vi "Create.vi"(8 "error in (no error)":errorcluster, 10 "Logging Rate":dbl) -> (0 "error out":errorcluster, 3 "Historian Logger out":refnum<class "Historian Logger.lvclass">)   [LabVIEW 2020, in "VolatusHistorian.lvlib" / "Historian Logger.lvclass"]
uses:
  Historian Logger.lvclass
  Historian Logger.lvclass/Historian Logger.ctl
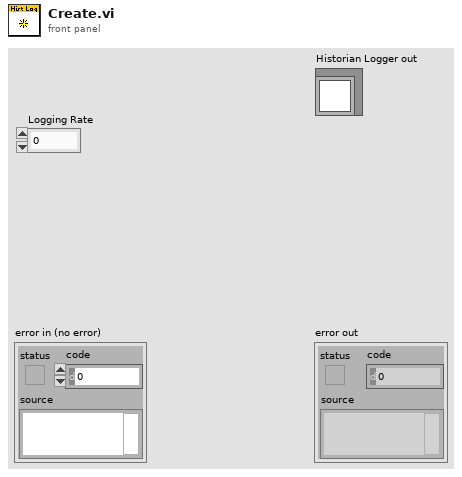
[diagram p1: front panel]
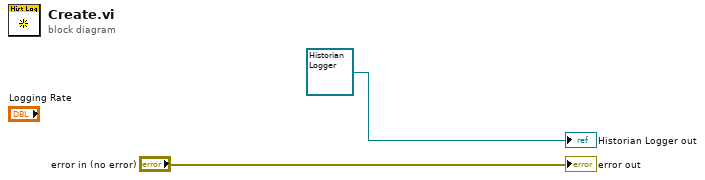
[diagram p0: block diagram]
diagram:
  "error out" <- "error in (no error)"
  "Historian Logger out" <- refnum<class "Historian Logger.lvclass"> refnum ("Historian Logger in")
